vi "Open Sample Container Connections.vi"(8 "error in (no error)":errorcluster, 11 "Container in":T1) -> (0 "error out":errorcluster, 3 "Container out":T1)   [LabVIEW 2015]
uses:
  Controls/Sample Container.ctl
  Sample/Sample.lvclass
  Sample/Sample.lvclass/Sample.ctl
  Sample/Mixed Sample.vi
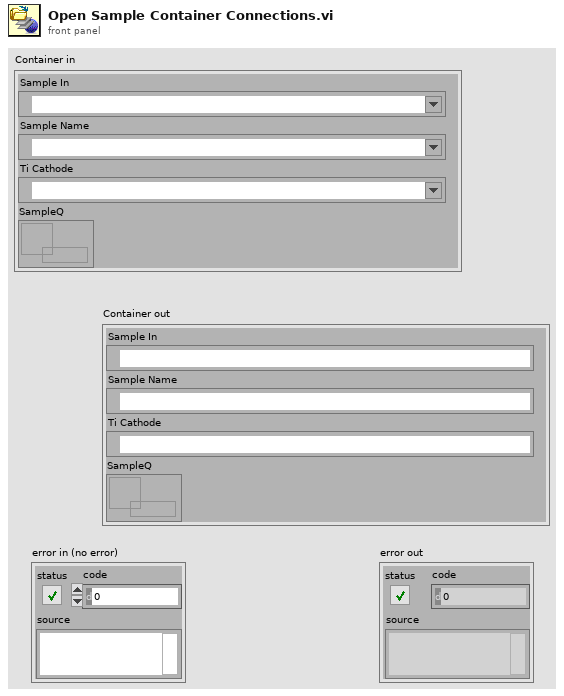
[diagram p1: front panel]
types:
  T1 = typedef "Sample Container.ctl" = cluster{"Sample In":refnum<k21>, "Sample Name":refnum<k21>, "Ti Cathode":refnum<k21>, "SampleQ":refnum<queue>}
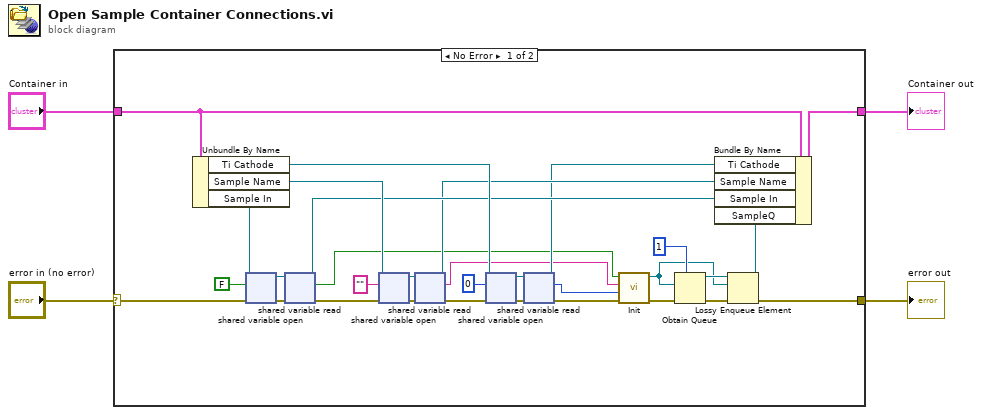
[diagram p0: block diagram]
diagram:
  n1 = case shown="No Error" "error in (no error)" {
    selector: "error in (no error)" -> [w35 w37]
    tunnel: "Container in" -> [w34 w36]
    tunnel: [w7 w37] -> w2
    tunnel: [w33 w36] -> w1
    frame No Error {
      n2 = Unbundle By Name(w34) -> ("Ti Cathode"=w27:refnum<k21>, "Sample Name"=w30:refnum<k21>, "Sample In"=w32:refnum<k21>)
      n3 = shared-variable-open(w32, w35, FALSE) -> (w25:refnum<k21>, w26:errorcluster)  [unwired: 1 in]
      n4 = shared-variable-read(w25, w26) -> (w24:refnum<k21>, w20:errorcluster, w14:bool)  [unwired: 1 out]
      n5 = shared-variable-open(w30, w20, "") -> (w22:refnum<k21>, w23:errorcluster)  [unwired: 1 in]
      n6 = shared-variable-read(w22, w23) -> (w21:refnum<k21>, w16:errorcluster, w13:string)  [unwired: 1 out]
      n7 = shared-variable-open(w27, w16, i8 0) -> (w18:refnum<k21>, w19:errorcluster)  [unwired: 1 in]
      n8 = shared-variable-read(w18, w19) -> (w17:refnum<k21>, w15:errorcluster, w12:i8)  [unwired: 1 out]
      n9 = call "Init.vi"("error in (no error)"=w15, "Ti Cathode"=w12, "Name"=w13, "Sample in"=w14) -> ("error out"=w11:errorcluster, "Sample out"=w5:refnum<class "Sample.lvclass">)  [unwired: 6 in]
      n10 = Obtain Queue(max queue size (-1, unlimited)=1, element data type=w5, error in (no error)=w11) -> (queue out=w8:refnum<queue>, error out=w10:errorcluster)  [unwired: 2 in, 1 out]
      n11 = Lossy Enqueue Element(queue=w8, element=w5, error in (no error)=w10) -> (queue out=w6:refnum<queue>, error out=w7:errorcluster)  [unwired: 2 out]
      n12 = Bundle By Name(cluster=w34, "Ti Cathode"=w17, "Sample Name"=w21, "Sample In"=w24, "SampleQ"=w6) -> (w33:T1)
    }
    frame Error {
    }
  }
  "error out" <- w2
  "Container out" <- w1
